vi "System_1.vi"() -> ()   [LabVIEW 2020]
doc: "Use this template to build a producer/consumer design pattern with events to produce queue items. Use this design pattern instead of the User Interface Event Handler pattern for user interfaces when you want to execute code asynchronously in response to an event without slowing the user interface responsiveness."
uses:
  <vilib>/Instr/_visa.llb/VISA Configure Serial Port (Instr).vi
panel:
  out "Input Voltage":dbl
  out "Motor Speed (RPM)":dbl
  in  "Motor Load":dbl(slide) scale=0.0..10.0
  in  "Initialize":bool
  out "Motor Speed":dbl(knob) scale=0.0..20.0
  out "Motor Torque":dbl(knob) scale=-50.0..20.0
  out "Input data":dbl
  in  "Baud rate (9600)":u32=9600
  in  "Serial Port Name":refnum<visa-resource-name>
  in  "Close":bool
  in  "Open":bool
  out "Connected":bool
  in  "stop":bool
  # "Motor simulation"
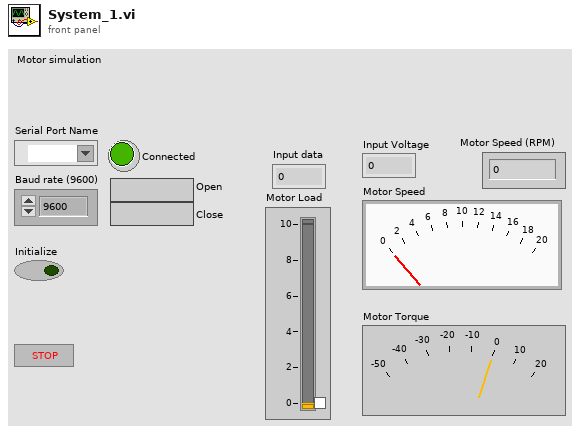
[diagram p1: front panel]
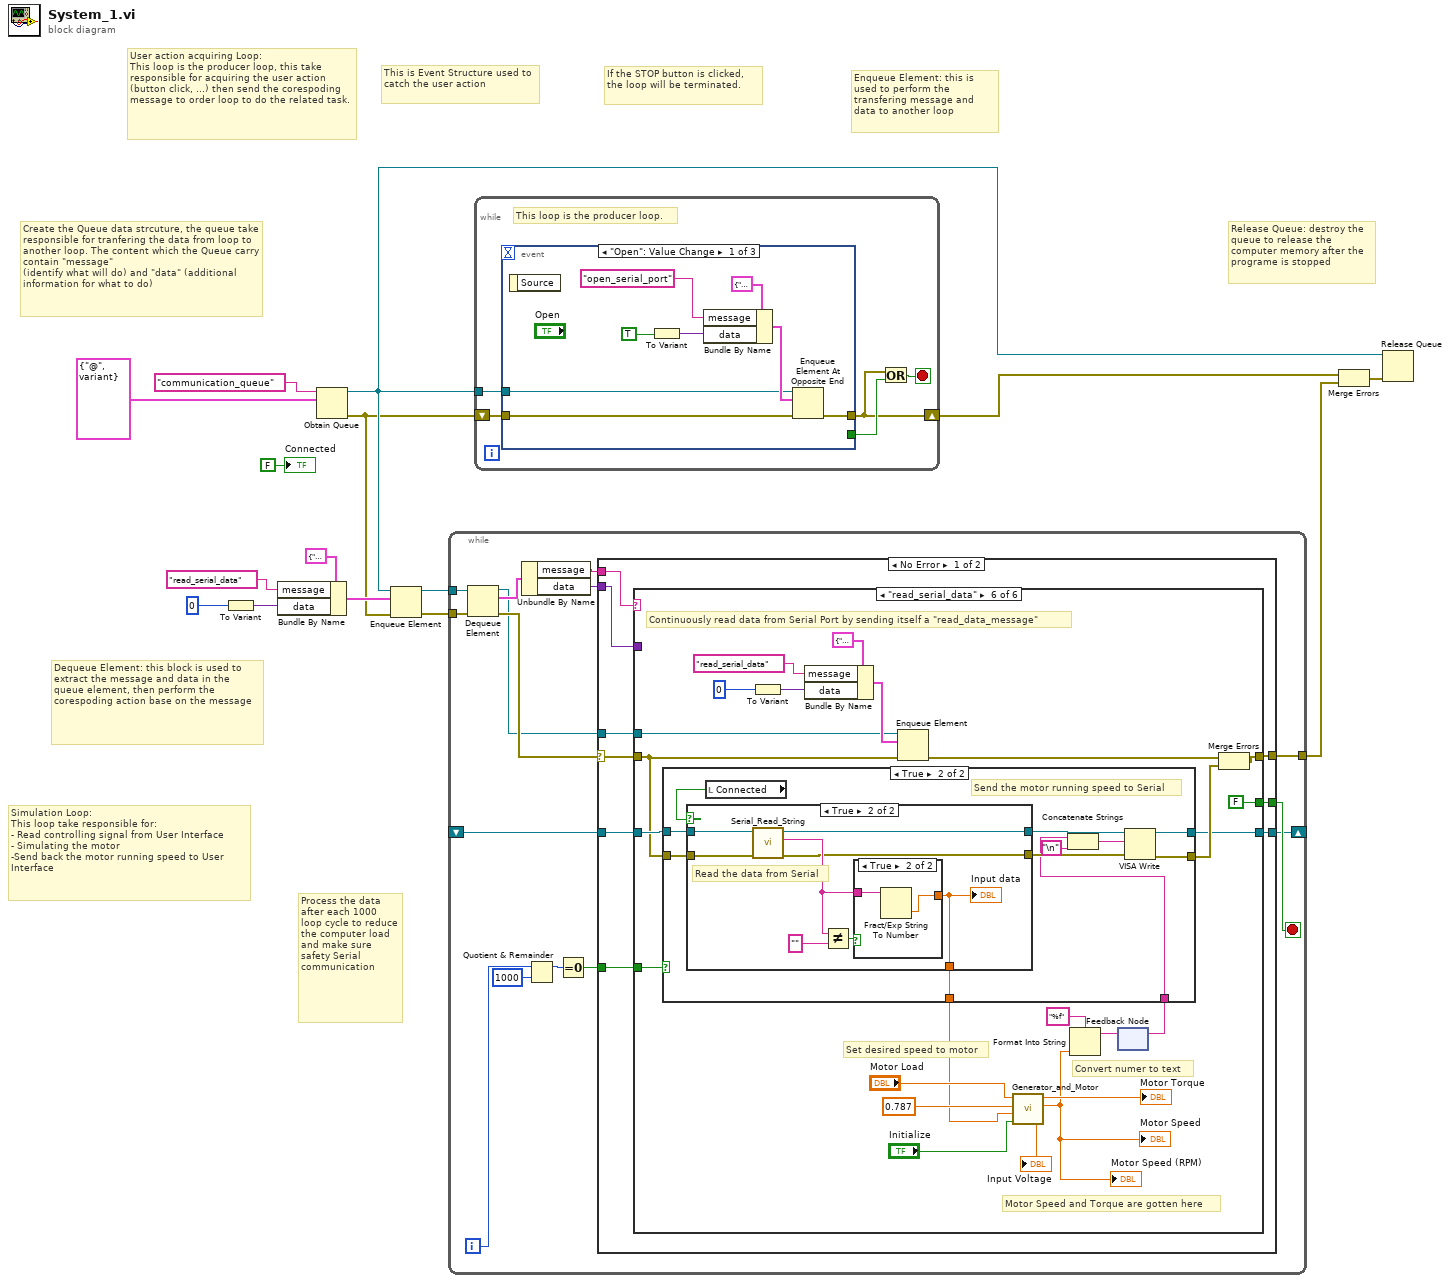
[diagram p0: block diagram]
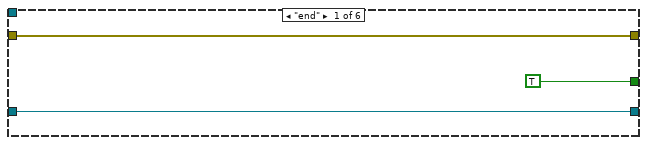
[diagram p2: hidden frame]
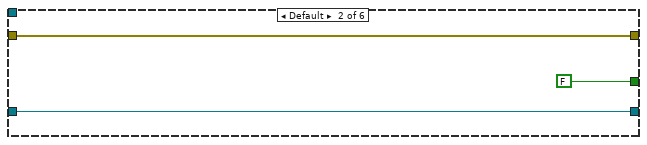
[diagram p3: hidden frame]
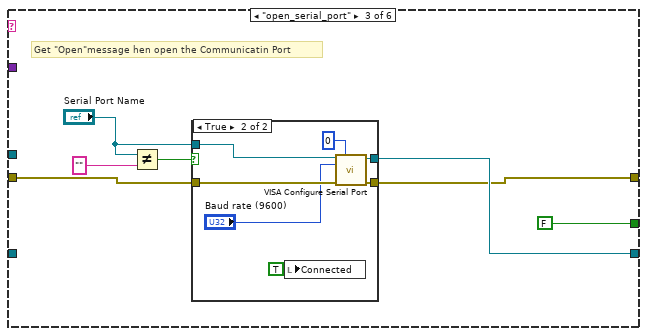
[diagram p4: hidden frame]
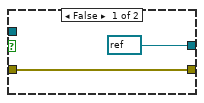
[diagram p5: hidden frame]
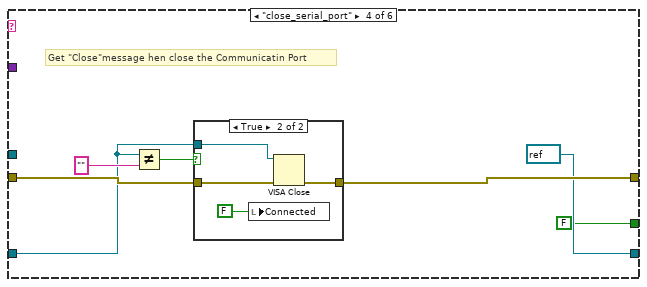
[diagram p6: hidden frame]
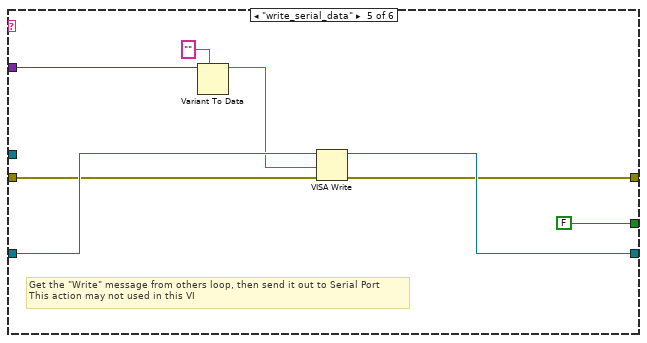
[diagram p8: hidden frame]
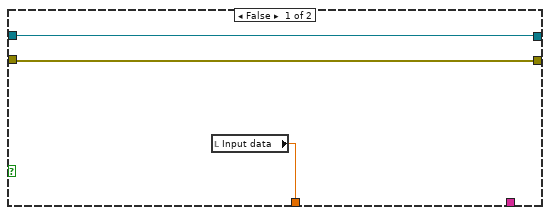
[diagram p9: hidden frame]
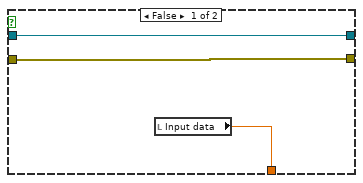
[diagram p10: hidden frame]
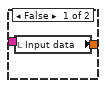
[diagram p11: hidden frame]
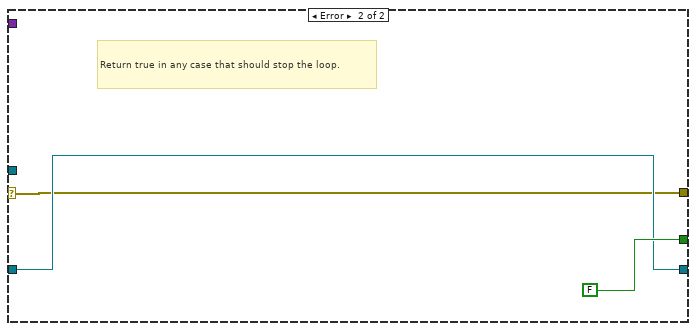
[diagram p12: hidden frame]
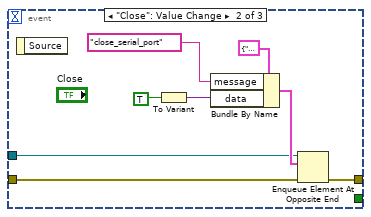
[diagram p13: hidden frame]
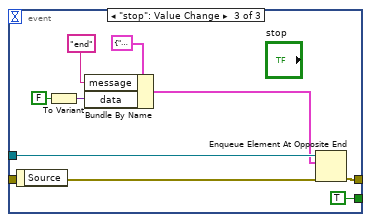
[diagram p14: hidden frame]
diagram:
  # "Process the data after each 1000 loop cycle to reduce the computer load and make sure safety Serial communication"
  # "Dequeue Element: this block is used to extract the message and data in the queue element, then perform the corespoding action base on the message"
  # "Simulation Loop:\nThis loop take responsible for: \n- Read controlling signal from User Interface\n- Simulating the motor\n-Send back the motor running speed to User Interface"
  # "Create the Queue data strcuture, the queue take responsible for tranfering the data from loop to another loop. The content which the Queue carry contain \"message\" \n(identify what will do) and \"data\" (additional information for what to do)"
  # "Release Queue: destroy the queue to release the computer memory after the programe is stopped"
  # "Enqueue Element: this is used to perform the transfering message and data to another loop"
  # "If the STOP button is clicked, the loop will be terminated."
  # "This is Event Structure used to catch the user action"
  # "User action acquiring Loop:\nThis loop is the producer loop, this take responsible for acquiring the user action (button click, ...) then send the corespoding message to order loop to do the related task."
  n1 = To Variant(anything=0) -> (Variant=w8:variant)
  n2 = Bundle By Name(cluster=cluster{"message":string, "data":variant} {"message"="@", "data"=variant}, "message"="read_serial_data", "data"=w8) -> (w11:cluster{"message":string, "data":variant})
  n3 = Obtain Queue(name (unnamed)="communication_queue", element data type=cluster{"message":string, "data":variant} {"message"="@", "data"=variant}) -> (queue out=w4:refnum<queue>, error out=w1:errorcluster)  [unwired: 3 in, 1 out]
  n4 = Enqueue Element(queue=w4, element=w11, error in (no error)=w1) -> (queue out=w5:refnum<queue>, error out=w6:errorcluster)  [unwired: 1 in, 1 out]
  n5 = while {
    tunnel: w5 -> [w30]
    tunnel: w6 -> [w26]
    shift-right: [w23] -> _
    shift-left: _ -> [w22]
    tunnel: [w21] -> w3
    i -> [w19]
    stop <- w28 stop-if-true
    n6 = Dequeue Element(queue=w30, error in (no error)=w26) -> (queue out=w20:refnum<queue>, element=w27:cluster{"message":string, "data":variant}, error out=w29:errorcluster)  [unwired: 1 in, 1 out]
    n7 = Unbundle By Name(w27) -> ("message"=w25:string, "data"=w24:variant)
    n8 = Quotient & Remainder(x=w19, y=1000) -> (x-y*floor(x/y)=w17:i32)  [unwired: 1 out]
    n9 = Equal To 0?(x=w17) -> (x = 0?=w16:bool)
    n10 = case shown="No Error" w29 {
      selector: w29 -> [w37 w134]
      tunnel: [w32 FALSE] -> w28
      tunnel: w25 -> [w39 _]
      tunnel: w24 -> [w38 _]
      tunnel: [w36 w135] -> w23
      tunnel: w22 -> [w35 w135]
      tunnel: [w34 w134] -> w21
      tunnel: w20 -> [w33 _]
      tunnel: w16 -> [w31 _]
      frame No Error {
        n11 = case shown="\"read_serial_data\"" w39 {
          tunnel: w38 -> [_ _ _ _ w75 _]
          tunnel: w37 -> [w41 w44 w52 w68 w80 w98]
          tunnel: [w42 w45 w48 refnum<visa-resource-name> refnum ("VISA resource name out") w79 w89] -> w36
          tunnel: w35 -> [w42 w45 _ w65 w81 w99]
          tunnel: [w41 w44 w47 w64 w78 w96] -> w34
          tunnel: w33 -> [_ _ _ _ _ w101]
          tunnel: [TRUE FALSE FALSE FALSE FALSE FALSE] -> w32
          tunnel: w31 -> [_ _ _ _ _ w88]
          frame "end" {
          }
          frame Default {
          }
          frame "open_serial_port" {
            # "Get \"Open\"message hen open the Communicatin Port"
            n12 = Not Equal?(x="Serial Port Name", y="") -> (x != y?=w50:bool)
            n13 = case shown="True" w50 {
              tunnel: w52 -> [w53 w60]
              tunnel: "Serial Port Name" -> [_ w57]
              tunnel: [refnum<visa-resource-name> refnum ("VISA resource name") w58] -> w48
              tunnel: [w53 w59] -> w47
              frame False {
              }
              frame True {
                n14 = local write "Connected"(TRUE ("Boolean")) -> ()
                n15 = call-poly "VISA Configure Serial Port"("VISA resource name"=w57, "timeout (10sec)"=u32 0, "baud rate (9600)"="Baud rate (9600)", "error in (no error)"=w60) -> ("VISA resource name out"=w58:refnum<visa-resource-name>, "error out"=w59:errorcluster)  [unwired: 10 in]
              }
            }
          }
          frame "close_serial_port" {
            # "Get \"Close\"message hen close the Communicatin Port"
            n16 = Not Equal?(x=w65, y="") -> (x != y?=w66:bool)
            n17 = case shown="True" w66 {
              tunnel: w68 -> [w69 w73]
              tunnel: w65 -> [_ w72]
              tunnel: [w69 w70] -> w64
              frame False {
              }
              frame True {
                n18 = local write "Connected"(FALSE ("Boolean")) -> ()
                n19 = VISA Close(VISA resource name=w72, error in (no error)=w73) -> (error out=w70:errorcluster)
              }
            }
          }
          frame "write_serial_data" {
            # "Get the \"Write\" message from others loop, then send it out to Serial Port\nThis action may not used in this VI"
            n20 = Variant To Data(type="", Variant=w75) -> (data=w74:string)  [unwired: 1 in, 1 out]
            n21 = VISA Write(VISA resource name=w81, write buffer=w74, error in (no error)=w80) -> (VISA resource name out=w79:refnum<visa-resource-name>, error out=w78:errorcluster)  [unwired: 1 out]
          }
          frame "read_serial_data" {
            # "Convert numer to text"
            # "Motor Speed and Torque are gotten here"
            # "Set desired speed to motor"
            # "Continuously read data from Serial Port by sending itself a \"read_data_message\""
            n22 = To Variant(anything=0) -> (Variant=w102:variant)
            n23 = Bundle By Name(cluster=cluster{"message":string, "data":variant} {"message"="@", "data"=variant}, "message"="read_serial_data", "data"=w102) -> (w105:cluster{"message":string, "data":variant})
            n24 = Enqueue Element(queue=w101, element=w105, error in (no error)=w98) -> (error out=w97:errorcluster)  [unwired: 1 in, 2 out]
            n25 = feedback #1() -> (w86:string)  [unwired: 1 in]
            n26 = case shown="True" w88 {
              tunnel: w99 -> [w107 w119]
              tunnel: w98 -> [w106 w118]
              tunnel: [w106 w114] -> w90
              tunnel: [w108 w113] -> w84
              tunnel: [w107 w112] -> w89
              tunnel: w86 -> [_ w110]
              frame False {
                n27 = local read "Input data"() -> (w108:dbl)
              }
              frame True {
                # "Send the motor running speed to Serial"
                n28 = local read "Connected"() -> (w117:bool)
                n29 = case shown="True" w117 {
                  tunnel: w119 -> [w122 w130]
                  tunnel: w118 -> [w121 w129]
                  tunnel: [w121 w124] -> w115
                  tunnel: [w122 w125] -> w116
                  tunnel: [w120 w123] -> w113
                  frame False {
                    n30 = local read "Input data"() -> (w120:dbl)
                  }
                  frame True {
                    # "Read the data from Serial"
                    n31 = call "Serial_Read_String.vi"("error in (no error)"=w129, "VISA Refnum in"=w130) -> ("error out"=w124:errorcluster, "read buffer"=w126:string, "VISA Refnum out"=w125:refnum<visa-resource-name>)  [unwired: 7 in]
                    n32 = Not Equal?(x=w126, y="") -> (x != y?=w127:bool)
                    n33 = case shown="True" w127 {
                      tunnel: w126 -> [_ w133]
                      tunnel: [w131 w132] -> w123
                      frame False {
                        n34 = local read "Input data"() -> (w131:dbl)
                      }
                      frame True {
                        n35 = Fract/Exp String To Number(string=w133) -> (number=w132:dbl)  [unwired: 3 in, 1 out]
                      }
                    }
                    "Input data" <- w123
                  }
                }
                n36 = Concatenate Strings(w110, "\n") -> (w109:string)
                n37 = VISA Write(VISA resource name=w116, write buffer=w109, error in (no error)=w115) -> (VISA resource name out=w112:refnum<visa-resource-name>, error out=w114:errorcluster)  [unwired: 1 out]
              }
            }
            n38 = call "Generator_and_Motor.vi"("Initialize"="Initialize", "Speed"=w84, "Speed Voltage Factor"=0.787, "Motor Load"="Motor Load") -> ("Voltage"=→"Input Voltage":dbl, "Motor Speed"=w83:dbl, "Motor Torque"=→"Motor Torque":dbl)  [unwired: 5 in]
            "Motor Speed" <- w83
            "Motor Speed (RPM)" <- w83
            n39 = Format Into String(format string="%f", w83) -> (resulting string=w87:string)  [unwired: 2 in, 1 out]
            n40 = feedback-in #1(w87) -> ()
            n41 = Merge Errors(w97, w90) -> (w96:errorcluster)
          }
        }
      }
      frame Error {
        # "Return true in any case that should stop the loop."
      }
    }
  }
  n42 = while {
    shift-right: [w138] -> w12
    shift-left: w1 -> [w141]
    tunnel: w4 -> [w137]
    stop <- w139 stop-if-true
    # "This loop is the producer loop."
    n43 = event shown="[0] \"Open\": Value Change" {
      selector: _ -> [_ _ _]
      dyn-events: _ -> [_ _ _]
      timeout: _ -> [_ _ _]
      tunnel: w141 -> [w145 w153 w159]
      tunnel: [w144 w152 w164] -> w138
      tunnel: [_ _ TRUE ("stop")] -> w140
      tunnel: w137 -> [w143 w151 w163]
      event "Open": Value Change {
        n44 = event-data() -> ()  [unwired: 1 in, 1 out]
        n45 = To Variant(anything=TRUE ("Open")) -> (Variant=w146:variant)
        n46 = Bundle By Name(cluster=cluster{"message":string, "data":variant} {"message"="@", "data"=variant}, "message"="open_serial_port", "data"=w146) -> (w149:cluster{"message":string, "data":variant})
        n47 = Enqueue Element At Opposite End(queue=w143, element=w149, error in (no error)=w145) -> (error out=w144:errorcluster)  [unwired: 1 in, 2 out]
      }
      event "Close": Value Change {
        n48 = event-data() -> ()  [unwired: 1 in, 1 out]
        n49 = To Variant(anything=TRUE ("Close")) -> (Variant=w154:variant)
        n50 = Bundle By Name(cluster=cluster{"message":string, "data":variant} {"message"="@", "data"=variant}, "message"="close_serial_port", "data"=w154) -> (w157:cluster{"message":string, "data":variant})
        n51 = Enqueue Element At Opposite End(queue=w151, element=w157, error in (no error)=w153) -> (error out=w152:errorcluster)  [unwired: 1 in, 2 out]
      }
      event "stop": Value Change {
        n52 = event-data() -> ()  [unwired: 1 in, 1 out]
        n53 = To Variant(anything=FALSE ("stop")) -> (Variant=w165:variant)
        n54 = Bundle By Name(cluster=cluster{"message":string, "data":variant} {"message"="@", "data"=variant}, "message"="end", "data"=w165) -> (w161:cluster{"message":string, "data":variant})
        n55 = Enqueue Element At Opposite End(queue=w163, element=w161, error in (no error)=w159) -> (error out=w164:errorcluster)  [unwired: 1 in, 2 out]
      }
    }
    n56 = Or(x=w138, y=w140) -> (x .or. y?=w139:bool)
  }
  n57 = Merge Errors(w12, w3) -> (w2:errorcluster)
  n58 = Release Queue(queue=w4, error in (no error)=w2) -> ()  [unwired: 1 in, 3 out]
  "Connected" <- FALSE ("Boolean")
